vi "Framework Test.vi"() -> ()   [LabVIEW 2017]
uses:
  Builds/Data Sharing Framework/Current/Core/DSF Core.lvlibp/Classes/Framework/Framework Options.ctl
  Builds/Data Sharing Framework/Current/Core/DSF Core.lvlibp/Typedefs/DSF FIFO Options.ctl
  Builds/Data Sharing Framework/Current/Core/DSF Core.lvlibp/Classes/Thread/DSF Thread Options.ctl
  Builds/Data Sharing Framework/Current/Core/DSF Core.lvlibp/Typedefs/DSF Plugin Options.ctl
  Builds/Data Sharing Framework/Current/Core/DSF Core.lvlibp/Typedefs/DSF Performance Options.ctl
  Builds/Data Sharing Framework/Current/Core/DSF Core.lvlibp/Typedefs/DSF Engine Framework Configuration.ctl
  Builds/Data Sharing Framework/Current/Core/DSF Core.lvlibp/Typedefs/DSF Engine Plugin Configuration.ctl
  Builds/Data Sharing Framework/Current/Core/DSF Core.lvlibp/Typedefs/DSF Timing Info.ctl
  Builds/Data Sharing Framework/Current/Core/DSF Core.lvlibp/Typedefs/DSF Engine Plugin Thread Configuration.ctl
  Builds/Data Sharing Framework/Current/Core/DSF Core.lvlibp/Typedefs/DSF Settings Info.ctl
  Builds/Data Sharing Framework/Current/Core/DSF Core.lvlibp/Typedefs/DSF Engine Transfer Group Configuration.ctl
  Builds/Data Sharing Framework/Current/Core/DSF Core.lvlibp/Typedefs/DSF Direction.ctl
  Builds/Data Sharing Framework/Current/Core/DSF Core.lvlibp/Typedefs/DSF Engine Transfer Configuration.ctl
  Builds/Data Sharing Framework/Current/Core/DSF Core.lvlibp/Typedefs/DSF Byte Order.ctl
  Builds/Data Sharing Framework/Current/Core/DSF Core.lvlibp/Typedefs/DSF Engine Channel Configuration.ctl
  Builds/Data Sharing Framework/Current/Core/DSF Core.lvlibp/Typedefs/DSF Data Type.ctl
  Builds/Data Sharing Framework/Current/Core/DSF Core.lvlibp/Typedefs/DSF Timeout Behavior.ctl
  <vilib>/Platform/TimedLoop/XDataNode/timing_clust.ctl
  <vilib>/Platform/TimedLoop/XDataNode/nitl_modes.ctl
  <vilib>/Platform/TimedLoop/XDataNode/wakeup.ctl
  Builds/Data Sharing Framework/Current/Core/DSF Core.lvlibp/Classes/Framework/Framework.lvclass
  <vilib>/NI/Memory Manager/Classes/Pointer/Pointer.lvclass/Pointer.ctl
  <vilib>/NI/Memory Manager/Classes/Pointer/Read Bool.vi
  <vilib>/NI/Memory Manager/Classes/Pointer/Write Bool.vi
  <vilib>/NI/Memory Manager/Classes/Pointer/Set Address.vi
  <vilib>/NI/Memory Manager/Classes/Pointer/Set Size.vi
  <vilib>/NI/Memory Manager/Classes/Pointer/Set Internal.vi
  <vilib>/NI/Memory Manager/Classes/Pointer/Check Null Pointer.vi
  <vilib>/NI/Memory Manager/Classes/Pointer/Clear (No Check).vi
  <vilib>/NI/Memory Manager/Classes/Pointer/Write I32.vi
  <vilib>/NI/Memory Manager/Classes/Pointer/Read U32.vi
  <vilib>/NI/Memory Manager/Classes/Pointer/Write U32.vi
  <vilib>/NI/Memory Manager/Classes/Pointer/Read (No Check).vi
  <vilib>/NI/Memory Manager/Classes/Pointer/Read (No Check) Bool.vi
  <vilib>/NI/Memory Manager/Classes/Pointer/Check Move.vi
  <vilib>/NI/Memory Manager/Classes/Pointer/Write (No Check).vi
  <vilib>/NI/Memory Manager/Classes/Pointer/Write (No Check) Bool.vi
  <vilib>/NI/Memory Manager/Classes/Pointer/Read I32.vi
  <vilib>/NI/Memory Manager/Classes/Pointer/Errors.vi
  <vilib>/NI/Memory Manager/Classes/Pointer/Null Pointer.vi
  <vilib>/NI/Memory Manager/Classes/Pointer/Is Null.vi
  <vilib>/NI/Memory Manager/Classes/Pointer/Clear Subset (No Check).vi
  <vilib>/NI/Memory Manager/Classes/Pointer/Write (No Check) I32.vi
  <vilib>/NI/Memory Manager/Classes/Pointer/Read (No Check) U32.vi
  <vilib>/NI/Memory Manager/Classes/Pointer/Write (No Check) U32.vi
  <vilib>/NI/Memory Manager/Classes/Pointer/Check Count.vi
  <vilib>/NI/Memory Manager/Classes/Pointer/Check Bounds (Power of 2).vi
  <vilib>/NI/Memory Manager/Classes/Pointer/Read (No Check) I32.vi
  <vilib>/NI/Memory Manager/Classes/Pointer/Create Error.vi
  <vilib>/NI/Memory Manager/Classes/Pointer/Out of Bounds.vi
  <vilib>/NI/Memory Manager/Classes/Pointer/Check Bounds.vi
  <vilib>/NI/Memory Manager/VIs/New Error Cluster Constant.vi
  <vilib>/NI/Memory Manager/VIs/New Error Cluster Constant (512B).vi
  <vilib>/NI/Memory Manager/VIs/Error Cluster.Set Status.vi
  <vilib>/NI/Memory Manager/VIs/Error Cluster.Set Code.vi
  <vilib>/NI/Memory Manager/VIs/Error Cluster.Set VI Source.vi
  <vilib>/NI/Memory Manager/Constants/Constants.vi
  <vilib>/NI/Memory Manager/Constants/Library Name.vi
  <vilib>/NI/Memory Manager/Classes/Pointer/Pointer Error Info.vi
  <vilib>/NI/Memory Manager/VIs/Source.Write.String.vi
  <vilib>/NI/Memory Manager/Constants/Pointer Class Name.vi
  <vilib>/NI/Memory Manager/Classes/Pointer/Write Pointer Size.vi
  <vilib>/NI/Memory Manager/VIs/Source.Write.Scalar.Base10.vi
  <vilib>/NI/Memory Manager/VIs/Source.Write.Scalar.Base10 (U64).vi
  <vilib>/NI/Memory Manager/Classes/Pointer/Check Pointer Bounds.vi
  <vilib>/NI/Memory Manager/Classes/Pointer/Check Buffer Bounds.vi
  <vilib>/NI/Memory Manager/Classes/Pointer/Buffer Underflow.vi
  <vilib>/NI/Memory Manager/Classes/Pointer/Pointer.lvclass
  <vilib>/platform/TimedLoop/XDataNode/XDataNode.xnode
  <vilib>/Platform/TimedLoop/XDataNode/XDNodeRunTimeDep.lvlib
  Builds/Data Sharing Framework/Current/Core/DSF Core.lvlibp/Classes/Configuration/Configuration Session.lvclass
  Builds/Data Sharing Framework/Current/Core/DSF Core.lvlibp/Classes/Performance/Performance.lvclass
  Builds/Data Sharing Framework/Current/Core/DSF Core.lvlibp
  Builds/Data Sharing Framework/Current/Core/DSF Core.lvlibp/1abvi3w/vi.lib/NI/Memory Manager/Classes/Pointer/Pointer.lvclass
panel:
  in  "Components Directory":path=path "C:/Builds/Data Sharing Framework/Windows/32/Components"
  in  "Framework Configuration":T1={"Plugins"=[{"name"="UDP", "components"=["UDP", "String Type Converter"], "cycle timing"={"priority"=1000, "decimation"=10, "offset"=0}, "threads"=[{"buffer converter settings"=[], "transceiver settings"=[{"key"="Local Port", "value"="50000"}, {"key"="Local Address", "value"="localhost"}], "processor"=-2, "priority offset"=0}, {"buffer converter settings"=[], "transceiver settings"=[{"key"="Local Port", "value"="50001"}, {"key"="Local Address", "value"="localhost"}], "processor"=-2, "priority offset"=0}, {"buffer converter settings"=[], "transceiver settings"=[{"key"="Local Port", "value"="50002"}, {"key"="Local Address", "value"="localhost"}], "processor"=-2, "priority offset"=0}, {"buffer converter settings"=[], "transceiver settings"=[{"key"="Local Port", "value"="50003"}, {"key"="Local Address", "value"="localhost"}], "processor"=-2, "priority offset"=0}], "Transfer Groups"=[{"name"="Group0", "direction"=enum."Tx", "cycle timing"={"priority"=100, "decimation"=1, "offset"=0}, "thread index"=0, "settings"=[], "Transfers"=[{"name"="Transfer0", "byte order"=enum."big-endian", "settings"=[{"key"="Destination Address", "value"="localhost"}, {"key"="Destination Port", "value"="60000"}], "channels"=[{"string offset"=0, "string data type"=enum."Bool", "engine data type"=enum."DBL", "name"="Bool", "settings"=[], "units"="V"}, {"string offset"=1, "string data type"=enum."SGL", "engine data type"=enum."DBL", "name"="SGL", "settings"=[], "units"="V"}, {"string offset"=5, "string data type"=enum."DBL", "engine data type"=enum."DBL", "name"="DBL", "settings"=[], "units"="V"}, {"string offset"=13, "string data type"=enum."I8", "engine data type"=enum."DBL", "name"="I8", "settings"=[], "units"="V"}, {"string offset"=14, "string data type"=enum."I16", "engine data type"=enum."DBL", "name"="I16", "settings"=[], "units"="V"}, {"string offset"=16, "string data type"=enum."I32", "engine data type"=enum."DBL", "name"="I32", "settings"=[], "units"="V"}, {"string offset"=20, "string data type"=enum."I64", "engine data type"=enum."DBL", "name"="I64", "settings"=[], "units"="V"}, {"string offset"=28, "string data type"=enum."U8", "engine data type"=enum."DBL", "name"="U8", "settings"=[], "units"="V"}, {"string offset"=29, "string data type"=enum."U16", "engine data type"=enum."DBL", "name"="U16", "settings"=[], "units"="V"}, {"string offset"=31, "string data type"=enum."U32", "engine data type"=enum."DBL", "name"="U32", "settings"=[], "units"="V"}, {"string offset"=35, "string data type"=enum."U64", "engine data type"=enum."DBL", "name"="U64", "settings"=[], "units"="V"}]}], "timeout behavior"=enum."Increment Late Count"}, {"name"="Group1", "direction"=enum."Tx", "cycle timing"={"priority"=100, "decimation"=2, "offset"=0}, "thread index"=1, "settings"=[], "Transfers"=[{"name"="Transfer0", "byte order"=enum."big-endian", "settings"=[{"key"="Destination Address", "value"="localhost"}, {"key"="Destination Port", "value"="60001"}], "channels"=[{"string offset"=0, "string data type"=enum."Bool", "engine data type"=enum."DBL", "name"="Bool", "settings"=[], "units"="V"}, {"string offset"=1, "string data type"=enum."SGL", "engine data type"=enum."DBL", "name"="SGL", "settings"=[], "units"="V"}, {"string offset"=5, "string data type"=enum."DBL", "engine data type"=enum."DBL", "name"="DBL", "settings"=[], "units"="V"}, {"string offset"=13, "string data type"=enum."I8", "engine data type"=enum."DBL", "name"="I8", "settings"=[], "units"="V"}, {"string offset"=14, "string data type"=enum."I16", "engine data type"=enum."DBL", "name"="I16", "settings"=[], "units"="V"}, {"string offset"=16, "string data type"=enum."I32", "engine data type"=enum."DBL", "name"="I32", "settings"=[], "units"="V"}, {"string offset"=20, "string data type"=enum."I64", "engine data type"=enum."DBL", "name"="I64", "settings"=[], "units"="V"}, {"string offset"=28, "string data type"=enum."U8", "engine data type"=enum."DBL", "name"="U8", "settings"=[], "units"="V"}, {"string offset"=29, "string data type"=enum."U16", "engine data type"=enum."DBL", "name"="U16", "settings"=[], "units"="V"}, {"string offset"=31, "string data type"=enum."U32", "engine data type"=enum."DBL", "name"="U32", "settings"=[], "units"="V"}, {"string offset"=35, "string data type"=enum."U64", "engine data type"=enum."DBL", "name"="U64", "settings"=[], "units"="V"}]}], "timeout behavior"=enum."Increment Late Count"}, {"name"="Group2", "direction"=enum."Tx", "cycle timing"={"priority"=100, "decimation"=3, "offset"=0}, "thread index"=2, "settings"=[], "Transfers"=[{"name"="Transfer0", "byte order"=enum."big-endian", "settings"=[{"key"="Destination Address", "value"="localhost"}, {"key"="Destination Port", "value"="60002"}], "channels"=[{"string offset"=0, "string data type"=enum."Bool", "engine data type"=enum."DBL", "name"="Bool", "settings"=[], "units"="V"}, {"string offset"=1, "string data type"=enum."SGL", "engine data type"=enum."DBL", "name"="SGL", "settings"=[], "units"="V"}, {"string offset"=5, "string data type"=enum."DBL", "engine data type"=enum."DBL", "name"="DBL", "settings"=[], "units"="V"}, {"string offset"=13, "string data type"=enum."I8", "engine data type"=enum."DBL", "name"="I8", "settings"=[], "units"="V"}, {"string offset"=14, "string data type"=enum."I16", "engine data type"=enum."DBL", "name"="I16", "settings"=[], "units"="V"}, {"string offset"=16, "string data type"=enum."I32", "engine data type"=enum."DBL", "name"="I32", "settings"=[], "units"="V"}, {"string offset"=20, "string data type"=enum."I64", "engine data type"=enum."DBL", "name"="I64", "settings"=[], "units"="V"}, {"string offset"=28, "string data type"=enum."U8", "engine data type"=enum."DBL", "name"="U8", "settings"=[], "units"="V"}, {"string offset"=29, "string data type"=enum."U16", "engine data type"=enum."DBL", "name"="U16", "settings"=[], "units"="V"}, {"string offset"=31, "string data type"=enum."U32", "engine data type"=enum."DBL", "name"="U32", "settings"=[], "units"="V"}, {"string offset"=35, "string data type"=enum."U64", "engine data type"=enum."DBL", "name"="U64", "settings"=[], "units"="V"}]}], "timeout behavior"=enum."Increment Late Count"}, {"name"="Group3", "direction"=enum."Tx", "cycle timing"={"priority"=100, "decimation"=4, "offset"=0}, "thread index"=3, "settings"=[], "Transfers"=[{"name"="Transfer0", "byte order"=enum."big-endian", "settings"=[{"key"="Destination Address", "value"="localhost"}, {"key"="Destination Port", "value"="60003"}], "channels"=[{"string offset"=0, "string data type"=enum."Bool", "engine data type"=enum."DBL", "name"="Bool", "settings"=[], "units"="V"}, {"string offset"=1, "string data type"=enum."SGL", "engine data type"=enum."DBL", "name"="SGL", "settings"=[], "units"="V"}, {"string offset"=5, "string data type"=enum."DBL", "engine data type"=enum."DBL", "name"="DBL", "settings"=[], "units"="V"}, {"string offset"=13, "string data type"=enum."I8", "engine data type"=enum."DBL", "name"="I8", "settings"=[], "units"="V"}, {"string offset"=14, "string data type"=enum."I16", "engine data type"=enum."DBL", "name"="I16", "settings"=[], "units"="V"}, {"string offset"=16, "string data type"=enum."I32", "engine data type"=enum."DBL", "name"="I32", "settings"=[], "units"="V"}, {"string offset"=20, "string data type"=enum."I64", "engine data type"=enum."DBL", "name"="I64", "settings"=[], "units"="V"}, {"string offset"=28, "string data type"=enum."U8", "engine data type"=enum."DBL", "name"="U8", "settings"=[], "units"="V"}, {"string offset"=29, "string data type"=enum."U16", "engine data type"=enum."DBL", "name"="U16", "settings"=[], "units"="V"}, {"string offset"=31, "string data type"=enum."U32", "engine data type"=enum."DBL", "name"="U32", "settings"=[], "units"="V"}, {"string offset"=35, "string data type"=enum."U64", "engine data type"=enum."DBL", "name"="U64", "settings"=[], "units"="V"}]}], "timeout behavior"=enum."Increment Late Count"}], "settings"=[]}]}
  in  "Options":T13={"FIFO Options"={"Infinite Timeouts"=FALSE}, "Thread Options"={"Show FP On Call"=TRUE, "Close FP After Call"=TRUE, "Allow Debugging"=TRUE}, "Plugin Options"={"Default Components"=FALSE}, "Performance Options"={"Measure Period"=TRUE, "Measure Rx/Tx Duration"=TRUE}}
  in  "UDP Rx max size":i32=800
  in  "UDP Rx ports":u16[](array[numeric])=[60000, 60001, 60002, 60003]
  out "Framework Error":errorcluster
  out "Tx duration":u32 format="%d us"
  out "Rx duration":u32 format="%d us"
  out "Actual Frequency":dbl format="%.1pHz"
  in  "Configuration Path":path=path "C:/Users/Admin/Desktop/configuration.dsf"
  out "Framework Iteration":i32 format="%d cycles"
  out "Actual Period":u32 format="%d us"
  in  "Target PCL Period":u32=10000 caption="Target Period" format="%d us"
  in  "stop":bool
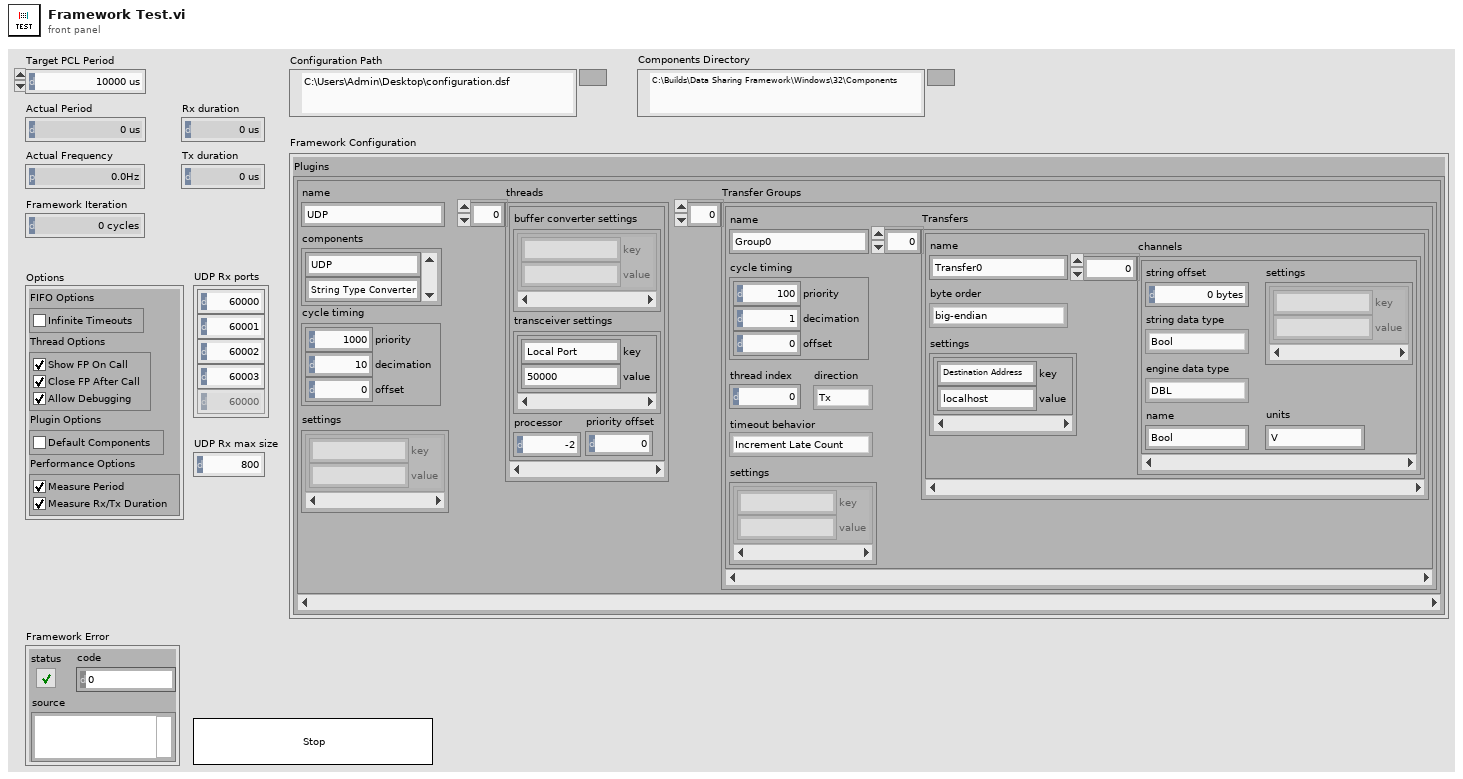
[diagram p1: front panel]
types:
  T1 = typedef "DSF Core.lvlibp/DSF Engine Framework Configuration.ctl" = cluster{"Plugins":T2[]}
  T2 = typedef "DSF Core.lvlibp/DSF Engine Plugin Configuration.ctl" = cluster{"name":string, "components":string[], "cycle timing":T3, "threads":T4[], "Transfer Groups":T6[], "settings":T5}
  T3 = typedef "DSF Core.lvlibp/DSF Timing Info.ctl" = cluster{"priority":u64, "decimation":u64, "offset":u64}
  T4 = typedef "DSF Core.lvlibp/DSF Engine Plugin Thread Configuration.ctl" = cluster{"buffer converter settings":T5, "transceiver settings":T5, "processor":i32, "priority offset":i16}
  T5 = typedef "DSF Core.lvlibp/DSF Settings Info.ctl" = cluster{"key":string, "value":string}[]
  T6 = typedef "DSF Core.lvlibp/DSF Engine Transfer Group Configuration.ctl" = cluster{"name":string, "direction":T7, "cycle timing":T3, "thread index":i32, "settings":T5, "Transfers":T8[], "timeout behavior":T12}
  T7 = typedef "DSF Core.lvlibp/DSF Direction.ctl" = enum8{"Tx", "Rx"}
  T8 = typedef "DSF Core.lvlibp/DSF Engine Transfer Configuration.ctl" = cluster{"name":string, "byte order":T9, "settings":T5, "channels":T10[]}
  T9 = typedef "DSF Core.lvlibp/DSF Byte Order.ctl" = enum8{"big-endian", "little-endian"}
  T10 = typedef "DSF Core.lvlibp/DSF Engine Channel Configuration.ctl" = cluster{"string offset":u64, "string data type":T11, "engine data type":T11, "name":string, "settings":T5, "units":string}
  T11 = typedef "DSF Core.lvlibp/DSF Data Type.ctl" = enum8{"Bool", "SGL", "DBL", "I8", "I16", "I32", "I64", "U8", "U16", "U32", "U64"}
  T12 = typedef "DSF Core.lvlibp/DSF Timeout Behavior.ctl" = enum8{"Increment Late Count", "Throw Error"}
  T13 = typedef "DSF Core.lvlibp/Framework.lvclass/Framework Options.ctl" = cluster{"FIFO Options":T14, "Thread Options":T15, "Plugin Options":T16, "Performance Options":T17}
  T14 = typedef "DSF Core.lvlibp/DSF FIFO Options.ctl" = cluster{"Infinite Timeouts":bool}
  T15 = typedef "DSF Core.lvlibp/DSF Thread Options.ctl" = cluster{"Show FP On Call":bool, "Close FP After Call":bool, "Allow Debugging":bool}
  T16 = typedef "DSF Core.lvlibp/DSF Plugin Options.ctl" = cluster{"Default Components":bool}
  T17 = typedef "DSF Core.lvlibp/DSF Performance Options.ctl" = cluster{"Measure Period":bool, "Measure Rx/Tx Duration":bool}
  T18 = typedef "User Interface Pointers.ctl" = cluster{"Stop":refnum<class "Pointer.lvclass">, "Iteration":refnum<class "Pointer.lvclass">, "Target Period":refnum<class "Pointer.lvclass">, "Actual Period":refnum<class "Pointer.lvclass">}
  T19 = typedef "XDNodeRunTimeDep.lvlib/timing_clust.ctl" = cluster{"Expected End [f-1]":u64, "Actual End [f-1]":u64, "Finished Late? [f-1]":bool, "Expected End [i-1]":u64, "Actual End [i-1]":u64, "Finished Late? [i-1]":bool, "Expected Start [i]":u64, "Actual Start [i]":u64, "Expected Start [f]":u64, "Actual Start [f]":u64, "Source Name":string, "Structure Name":string, "Period":i64, "Deadline":i64, "Offset":i64, "Start":i64, "Priority":i32, "Timeout":i32, "Mode":T20, "Wakeup Reason":T21, "Error":errorcluster, "Source Type":string, "Secondary Source Type":string, "Global End Time":u64, "Global Start Time":u64, "Frame Duration":u64, "Iteration Duration":u64, "Assigned CPU":i32, "I/O Scan Engine Mode":u32}
  T20 = typedef "XDNodeRunTimeDep.lvlib/nitl_modes.ctl" = enum32{"No Change", "Process missed periods, maintain original phase", "Discard missed periods, maintain original phase", "Process missed periods, ignore original phase", "Discard missed periods, ignore original phase"}
  T21 = typedef "XDNodeRunTimeDep.lvlib/wakeup.ctl" = enum32{"Normal", "Aborted", "Asynchronous wakeup", "Timing source error", "Timed loop error", "Timeout"}
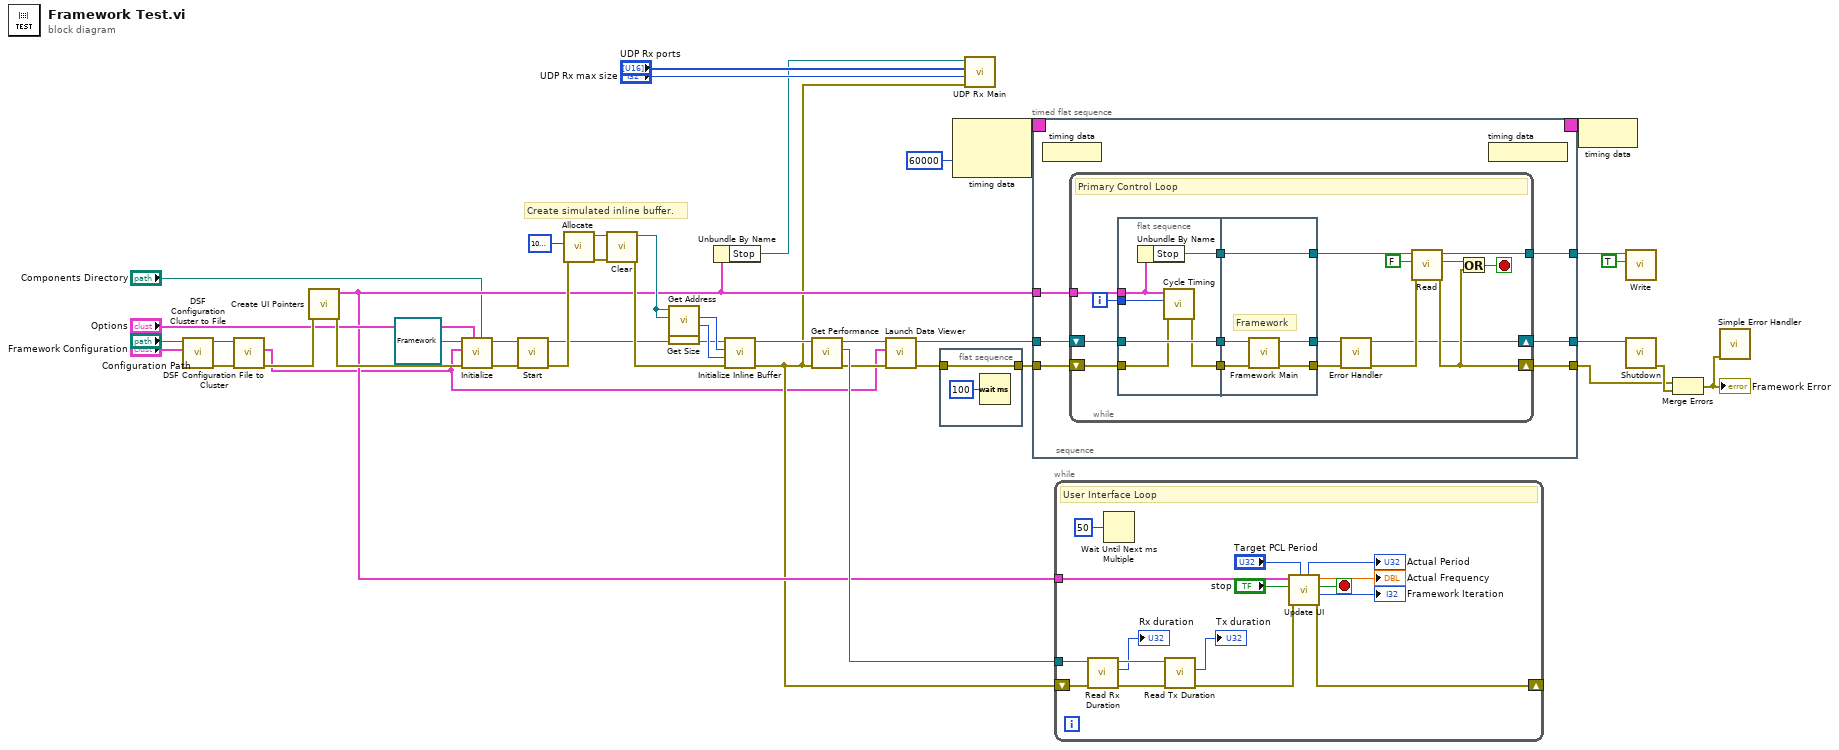
[diagram p0: block diagram]
diagram:
  # "Create simulated inline buffer."
  n1 = call "DSF Configuration Cluster to File.vi"("framework configuration"="Framework Configuration", "dsf configuration file path"="Configuration Path") -> ("error out"=w27:errorcluster, "dsf configuration file path dup"=w24:path)  [unwired: 8 in]
  n2 = call "DSF Configuration File to Cluster.vi"("error in (no error)"=w27, "dsf configuration file path"=w24) -> ("error out"=w21:errorcluster, "framework configuration out"=w2:T1)  [unwired: 7 in, 1 out]
  n3 = call "Create UI Pointers.vi"("error in (no error)"=w21) -> ("error out"=w20:errorcluster, "UI Pointers"=w7:T18)  [unwired: 9 in]
  n4 = call-dynamic "Initialize.vi"("components directory (default)"="Components Directory", "framework options"="Options", "error in (no error)"=w20, "framework configuration"=w2, "Framework in"=refnum<class "Framework.lvclass"> refnum) -> ("error out"=w10:errorcluster, "Framework out"=w11:refnum<class "Framework.lvclass">)  [unwired: 5 in]
  n5 = call-dynamic "Start.vi"("error in (no error)"=w10, "Framework in"=w11) -> ("error out"=w9:errorcluster, "Framework out"=w8:refnum<class "Framework.lvclass">)  [unwired: 8 in]
  n6 = call <vilib>:"Allocate.vi"("error in (no error)"=w9, "size"=u64 1000000 ("channel count")) -> ("error out"=w12:errorcluster, "Pointer out"=w14:refnum<class "Pointer.lvclass">)  [unwired: 8 in]
  n7 = call <vilib>:"Clear.vi"("error in (no error)"=w12, "Pointer in"=w14) -> ("error out"=w41:errorcluster, "Pointer out"=w13:refnum<class "Pointer.lvclass">)  [unwired: 8 in]
  n8 = call <vilib>:"Get Address.vi"("Pointer in"=w13) -> ("address"=w17:u64)  [unwired: 9 in, 1 out]
  n9 = call <vilib>:"Get Size.vi"("Pointer in"=w13) -> ("size"=w18:u64)  [unwired: 9 in, 1 out]
  n10 = Unbundle By Name(w7) -> ("Stop"=w28:refnum<class "Pointer.lvclass">)
  n11 = call "Initialize Inline Buffer.vi"("error in (no error)"=w41, "size"=w18, "address"=w17, "Framework in"=w8) -> ("error out"=w4:errorcluster, "Framework out"=w26:refnum<class "Framework.lvclass">)  [unwired: 6 in]
  n12 = call "Get Performance.vi"("Framework in"=w26) -> ("Performance"=w25:refnum<class "Performance.lvclass">, "Framework out"=w6:refnum<class "Framework.lvclass">)  [unwired: 9 in]
  n13 = call "Launch Data Viewer.vi"("error in (no error)"=w4, "Framework Configuration"=w2, "Framework in"=w6) -> ("error out"=w3:errorcluster, "Framework out"=w5:refnum<class "Framework.lvclass">)  [unwired: 7 in]
  n14 = flat-sequence {
    tunnel: [w43] -> w16
    tunnel: w3 -> [w43]
    frame #0 {
      n15 = Wait (ms)(milliseconds to wait=u32 100) -> ()  [unwired: 1 out]
    }
  }
  n16 = node-c288(60000 ("Priority")) -> (w40:T19)  [unwired: 1 in]
  n17 = call "UDP Rx Main.vi"("error in (no error)"=w4, "max size (800)"="UDP Rx max size", "ports"="UDP Rx ports", "Stop Pointer"=w28) -> ()  [unwired: 7 in, 1 out]
  n18 = timed-sequence {
    timing: w40 -> [_]
    timing-out: [_] -> w39
    tunnel: w5 -> [w49]
    tunnel: w16 -> [w48]
    tunnel: [w47] -> w36
    tunnel: [w46] -> w33
    tunnel: [w45] -> w38
    tunnel: w7 -> [w44]
    n19 = timed-flat-sequence {
      tunnel: w49 -> [w55]
      tunnel: w48 -> [w54]
      tunnel: [w53] -> w47
      tunnel: [w52] -> w46
      tunnel: [w51] -> w45
      tunnel: w44 -> [w50]
      n20 = node-c288() -> ()  [unwired: 1 in]
      n21 = while {
        shift-right: [w60] -> w53
        shift-left: w55 -> [w71]
        shift-right: [w69] -> w52
        shift-left: w54 -> [w72]
        tunnel: [w64] -> w51
        tunnel: w50 -> [w56]
        i -> [w57]
        stop <- w68 stop-if-true
        # "Primary Control Loop"
        n22 = flat-sequence {
          tunnel: w72 -> [w77]
          tunnel: w71 -> [w78]
          tunnel: [w76] -> w67
          tunnel: [w78] -> w66
          tunnel: [w73] -> w65
          tunnel: w57 -> [w75]
          tunnel: w56 -> [w74]
          tunnel: [w83] -> w70
          tunnel: [w82] -> w62
          tunnel: [w81] -> w63
          tunnel: w65 -> [w83]
          tunnel: w66 -> [w80]
          tunnel: w67 -> [w79]
          frame #0 {
            n23 = Unbundle By Name(w74) -> ("Stop"=w73:refnum<class "Pointer.lvclass">)
            n24 = call "Cycle Timing.vi"("error in (no error)"=w77, "iteration"=w75, "UI Pointers"=w74) -> ("error out"=w76:errorcluster)  [unwired: 8 in]
          }
          frame #1 {
            # "Framework"
            n25 = call "Framework Main.vi"("error in (no error)"=w79, "Framework in"=w80) -> ("error out"=w81:errorcluster, "Framework out"=w82:refnum<class "Framework.lvclass">)  [unwired: 8 in]
          }
        }
        n26 = call "Error Handler.vi"("error in (no error)"=w63, "Framework in"=w62) -> ("error out"=w61:errorcluster, "Framework out"=w60:refnum<class "Framework.lvclass">)  [unwired: 8 in]
        n27 = call-poly <vilib>:"Read.vi"("error in (no error)"=w61, "value in"=FALSE, "Pointer in"=w70) -> ("error out"=w69:errorcluster, "value out"=w59:bool, "Pointer out"=w64:refnum<class "Pointer.lvclass">)  [unwired: 5 in, 1 out]
        n28 = Or(x=w59, y=w69) -> (x .or. y?=w68:bool)
      }
      n29 = node-c288() -> ()  [unwired: 1 out]
    }
  }
  n30 = while {
    shift-right: [w87] -> _
    shift-left: w4 -> [w97]
    tunnel: w7 -> [w95]
    tunnel: w25 -> [w86]
    stop <- w93 stop-if-true
    # "User Interface Loop"
    n31 = call "Read Rx Duration.vi"("error in (no error)"=w97, "Framework Performance in"=w86) -> ("error out"=w96:errorcluster, "rx duration"=→"Rx duration":u32, "Framework Performance out"=w100:refnum<class "Performance.lvclass">)  [unwired: 7 in]
    n32 = Wait Until Next ms Multiple(millisecond multiple=u32 50 ("milliseconds to wait")) -> ()  [unwired: 1 out]
    n33 = call "Read Tx Duration.vi"("error in (no error)"=w96, "Framework Performance in"=w100) -> ("error out"=w88:errorcluster, "tx duration"=→"Tx duration":u32)  [unwired: 7 in, 1 out]
    n34 = call "Update UI.vi"("Target PCL Period"="Target PCL Period", "error in (no error)"=w88, "stop"="stop", "UI Pointers"=w95) -> ("error out"=w87:errorcluster, "Framework Iteration"=→"Framework Iteration":i32, "stop?"=w93:bool, "Actual Frequency"=→"Actual Frequency":dbl, "Actual Period"=→"Actual Period":u32)  [unwired: 3 in]
  }
  n35 = node-c288(w39) -> ()
  n36 = call-poly <vilib>:"Write.vi"("value"=TRUE, "Pointer in"=w38) -> ()  [unwired: 6 in, 4 out]
  n37 = call-dynamic "Shutdown.vi"("Framework in"=w36) -> ("error out"=w34:errorcluster)  [unwired: 9 in, 1 out]
  n38 = Merge Errors(w33, w34) -> (w32:errorcluster)
  "Framework Error" <- w32
  n39 = call <vilib>:"Simple Error Handler.vi"("error in (no error)"=w32) -> ()  [unwired: 4 in, 5 out]
